vi "Untitled 1.vi"() -> ()   [LabVIEW 2020]
panel:
  out "output variable":dbl
  out "Wykres V(t)":dbl(graph)
  out "V(t)":dbl
  out "h":dbl
  out "Qin":dbl format="%#_7g"
  out "time":dbl format="%#_5g"
  in  "Qin":dbl(slide) scale=0.0..10.0
  out "Wykres h(t)":dbl(graph)
  in  "Stop Button":bool
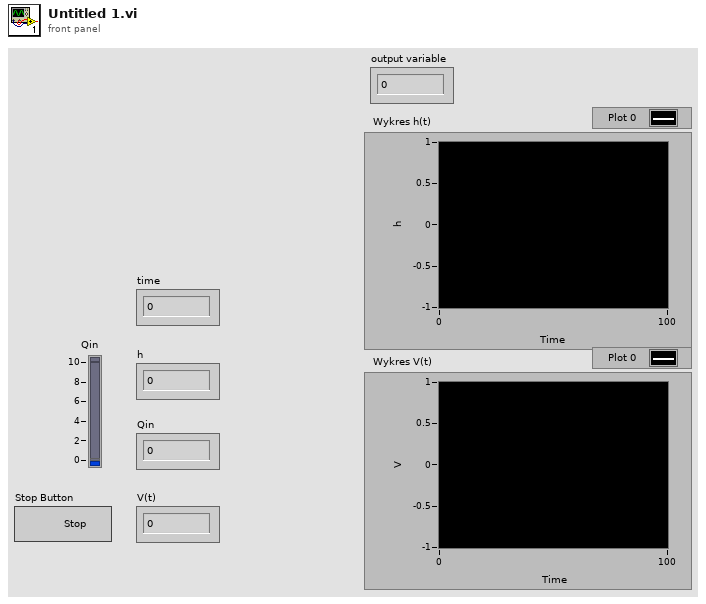
[diagram p1: front panel]
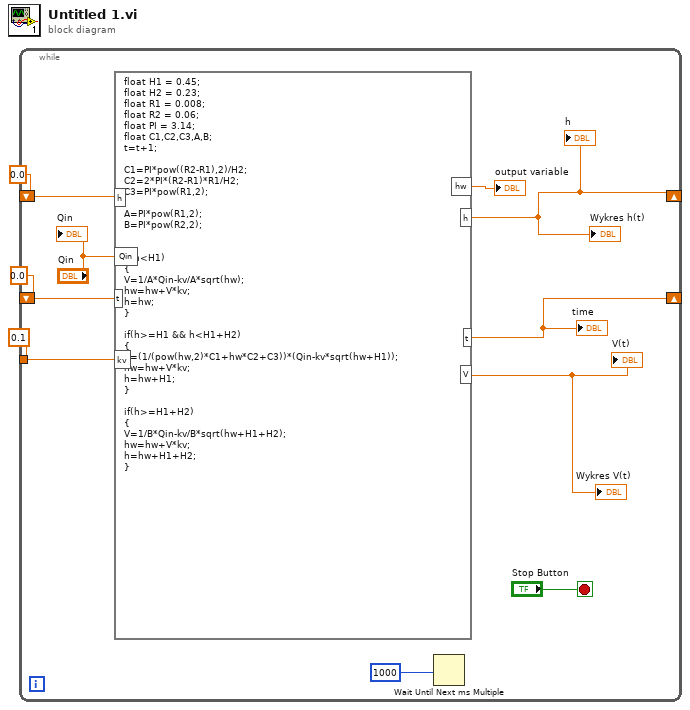
[diagram p0: block diagram]
diagram:
  n1 = while {
    shift-right: [w12] -> _
    shift-left: 0.0 -> [w11]
    shift-right: [w7] -> _
    shift-left: 0.0 ("t") -> [w9]
    tunnel: 0.1 ("input variable") -> [w6]
    stop <- "Stop Button" stop-if-true
    n2 = formula code="float H1 = 0.45;\nfloat H2 = 0.23;\nfloat R1 = 0.008;\nfloat R2 = 0.06;\nfloat PI = 3.14;\nfloat C1,C2,C3,A,B;\nt=t+1;\n\nC1=PI*pow((R2-R1),2)/H2;\nC2=2*PI*(R2-R1)*R1/H2;\nC3=PI*pow(R1,2);\n\nA=PI*pow(R1,2);\nB=PI*pow(R2,2);\n\n \nif(h<H1)\n{\nV=1/A*Qin-kv/A*sqrt(hw);\nhw=hw+V*kv;\nh=hw;\n}\n\nif(h>=H1 && h<H1+H2)\n{\nV=(1/(pow(hw,2)*C1+hw*C2+C3))*(Qin-kv*sqrt(hw+H1));\nhw=hw+V*kv;\nh=hw+H1;\n}\n\nif(h>=H1+H2)\n{\nV=1/B*Qin-kv/B*sqrt(hw+H1+H2);\nhw=hw+V*kv;\nh=hw+H1+H2;\n}"("Qin"="Qin", "h"=w11, "t"=w9, "kv"=w6) -> ("h"=w12:dbl, "t"=w7:dbl, "V"=→"V(t)" →"Wykres V(t)":dbl, "hw"=→"output variable":dbl)
    "Wykres h(t)" <- w12
    "time" <- w7
    "h" <- w12
    n3 = Wait Until Next ms Multiple(millisecond multiple=u32 1000) -> ()  [unwired: 1 out]
    "Qin" <- "Qin"
  }
